vi "Setting.vi"() -> ()   [LabVIEW 2020]
uses:
  Global_Variable/Global.vi
  <userlib>/_MGI/1D Array/MGI Average/MGI Average (DBL[]).vi
  Libraries/S7/S7.lvlib
panel:
  in  "速度":sgl format="%#_3f °/S"
  out "退出":bool=TRUE
  in  "STEP":string
  in  "工位二标定":bool
  in  "停止":bool
  in  "工位一标定":bool
  out "标定曲线":cluster{dbl[], dbl[]}[](graph)
  # "配置标定"
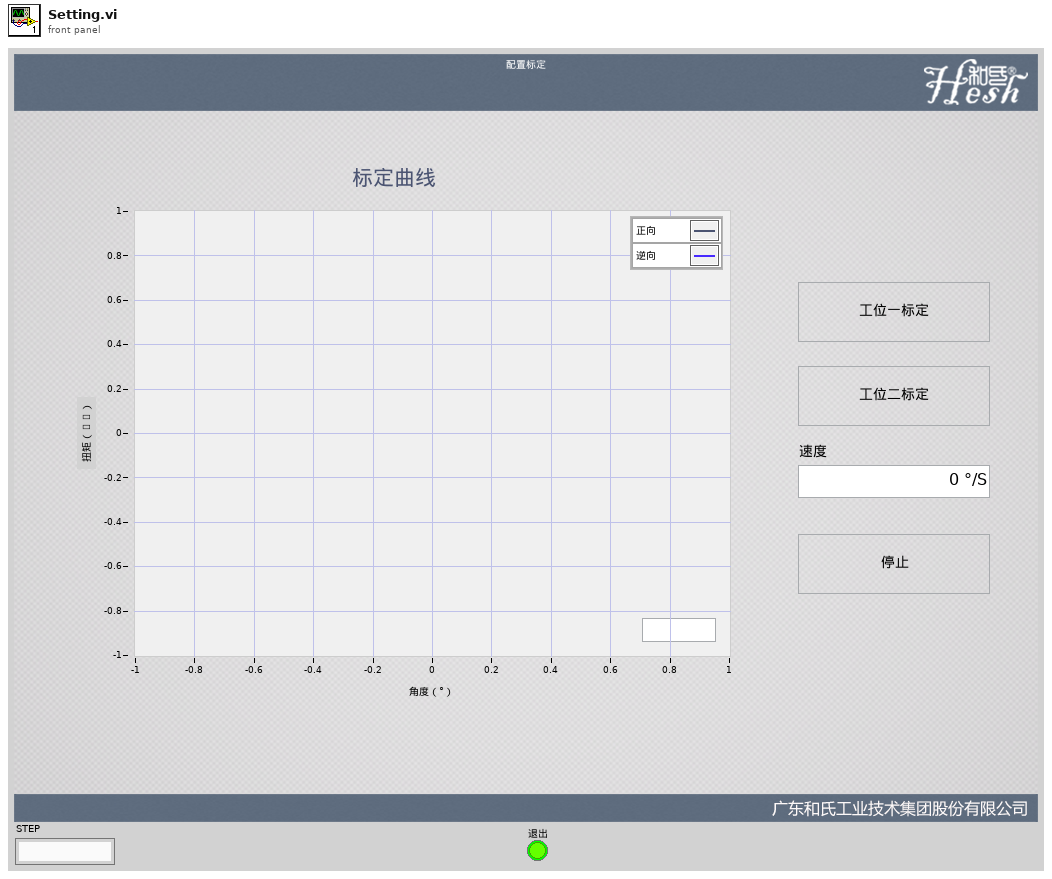
[diagram p1: front panel]
types:
  T1 = cluster{"工位一驱动伺服位移":sgl, "工位二驱动伺服位移":sgl, "工位一移载伺服位移":sgl, "工位二移载伺服位移":sgl, "工位一编码器位移":sgl, "工位二编码器位移":sgl, "工位一扭矩":sgl, "工位二扭矩":sgl}
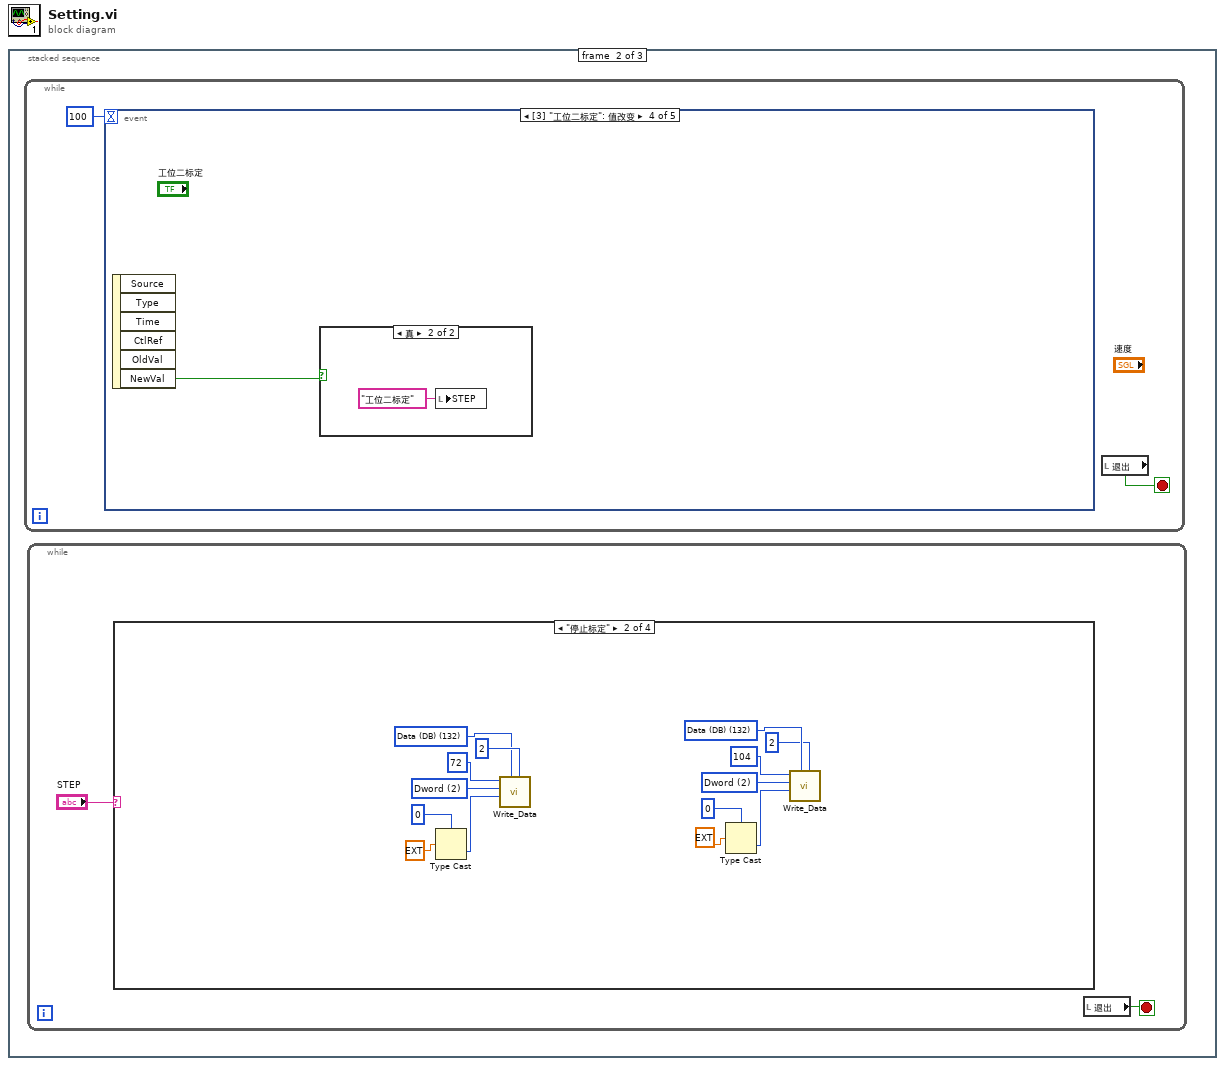
[diagram p0: block diagram]
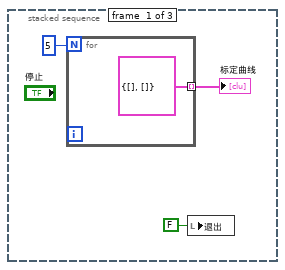
[diagram p2: hidden frame]
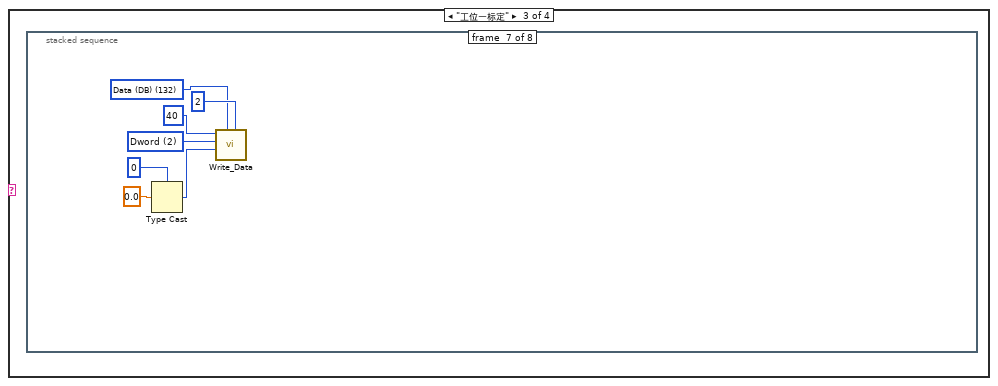
[diagram p4: hidden frame]
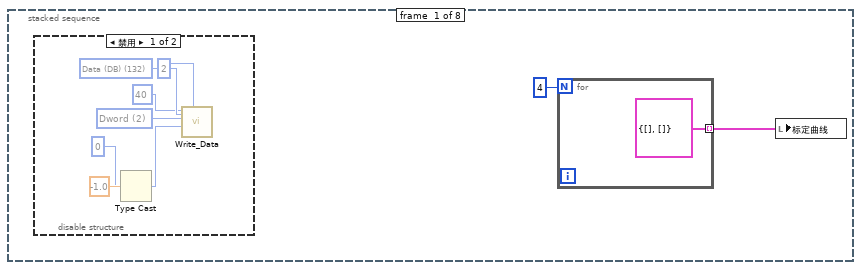
[diagram p5: hidden frame]
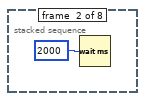
[diagram p7: hidden frame]
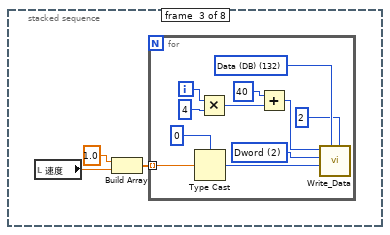
[diagram p8: hidden frame]
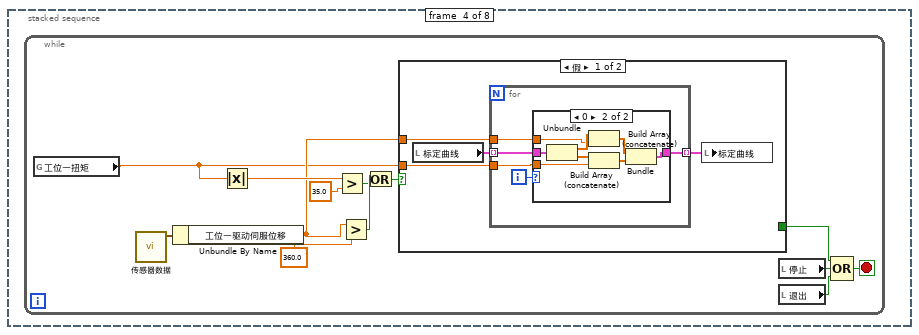
[diagram p9: hidden frame]
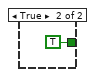
[diagram p11: hidden frame]
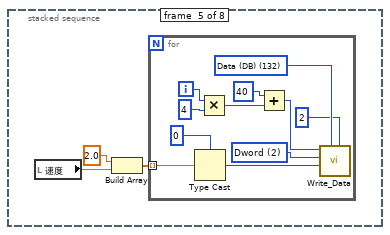
[diagram p12: hidden frame]
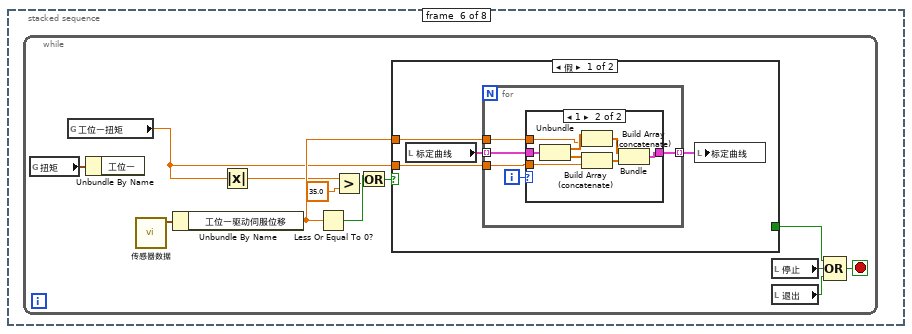
[diagram p13: hidden frame]
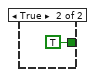
[diagram p15: hidden frame]
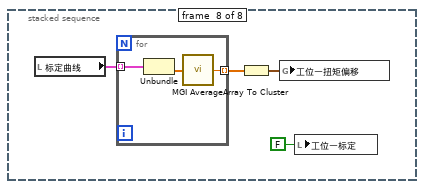
[diagram p16: hidden frame]
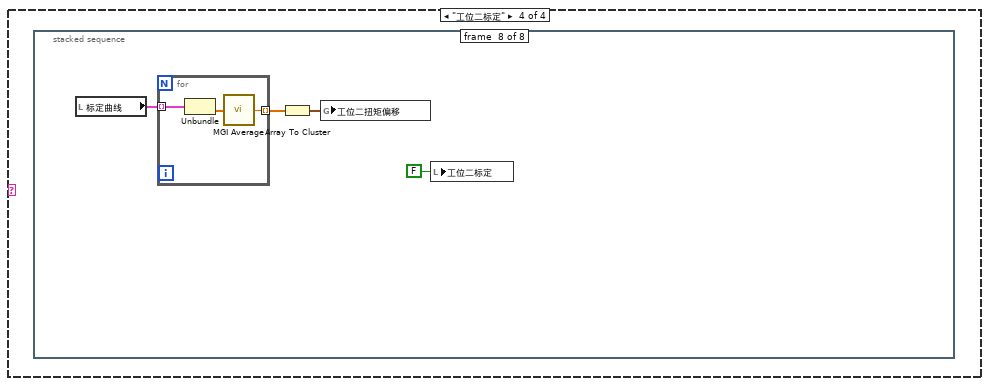
[diagram p17: hidden frame]
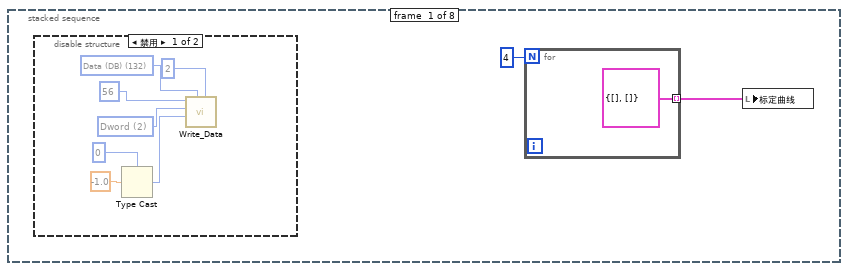
[diagram p18: hidden frame]
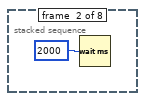
[diagram p20: hidden frame]
diagram:
  n1 = stacked-sequence {
    frame #0 {
      n2 = for {
        N: 5 -> [_]
        tunnel: [cluster{dbl[], dbl[]} {[], []}] -> w2 mode=indexing
      }
      "标定曲线" <- w2
      n3 = local write "退出"(FALSE ("退出")) -> ()
    }
    frame #1 {
      n4 = while {
        stop <- w256 stop-if-true
        n5 = event shown="[3] \"工位二标定\": 值改变" {
          selector: _ -> [_ _ _ _ _]
          dyn-events: _ -> [_ _ _ _ _]
          timeout: 100 -> [_ _ _ _ _]
          event Timeout {
            n6 = event-data() -> ()  [unwired: 1 in, 3 out]
          }
          event "工位一标定": Value Change {
            n7 = event-data() -> ("NewVal"=w258:bool)  [unwired: 1 in, 2 out]
            n8 = case shown="真" w258 {
              frame False {
              }
              frame True {
                n9 = local write "STEP"("工位一标定" ("STEP")) -> ()
              }
            }
          }
          event "停止": Value Change {
            n10 = event-data() -> ()  [unwired: 1 in, 4 out]
            n11 = local write "STEP"("停止标定" ("STEP")) -> ()
          }
          event "工位二标定": Value Change {
            n12 = event-data() -> ("NewVal"=w261:bool)  [unwired: 1 in, 5 out]
            n13 = case shown="真" w261 {
              frame False {
              }
              frame True {
                n14 = local write "STEP"("工位二标定" ("STEP")) -> ()
              }
            }
          }
          event Panel Close {
            n15 = event-data() -> ()  [unwired: 1 in, 4 out]
            n16 = global read "Global.vi" "产品型号"() -> (w264:string)
            n17 = call "标定数据保存.vi"("Section"=w264, "枚举"=enum16{"读取", "保存"}."保存") -> ()  [unwired: 10 in]
            "退出" <- TRUE ("退出")
          }
        }
        n18 = local read "退出"() -> (w256:bool)
      }
      n19 = while {
        stop <- w5 stop-if-true
        n20 = case shown="\"停止标定\"" "STEP" {
          frame "假", Default {
          }
          frame "停止标定" {
            w10 = u16 2 items=["byte", "word", "Dword"] ("数据类型")
            w12 = u8 132 items=["I/O (P)"=128, "Input (I)"=129, "Output (Q)"=130, "Bit Memory (M)"=131, "Data (DB)"=132, "Instance Data (DI)"=133, "Local Data (L)"=134, "Predecessor Local Data (VL)"=135] ("寄存器类型")
            w17 = u16 2 items=["byte", "word", "Dword"] ("数据类型")
            w15 = u8 132 items=["I/O (P)"=128, "Input (I)"=129, "Output (Q)"=130, "Bit Memory (M)"=131, "Data (DB)"=132, "Instance Data (DI)"=133, "Local Data (L)"=134, "Predecessor Local Data (VL)"=135] ("寄存器类型")
            n21 = Type Cast(type=u32 0, x=ext 0.0) -> (*(type *) &x=w19:u32)
            n22 = call "Write_Data.vi"("DB #"=u16 2, "寄存器类型"=w15, "写入数据"=w19, "数据类型"=w17, "写入地址"=u32 72) -> ()  [unwired: 4 in, 3 out]
            n23 = Type Cast(type=u32 0, x=ext 0.0) -> (*(type *) &x=w8:u32)
            n24 = call "Write_Data.vi"("DB #"=u16 2, "寄存器类型"=w12, "写入数据"=w8, "数据类型"=w10, "写入地址"=u32 104) -> ()  [unwired: 4 in, 3 out]
          }
          frame "工位一标定" {
            n25 = stacked-sequence {
              frame #0 {
                n26 = disable-structure shown="禁用" {
                  frame Disabled {
                    w26 = u16 2 items=["byte", "word", "Dword"] ("数据类型")
                    w28 = u8 132 items=["I/O (P)"=128, "Input (I)"=129, "Output (Q)"=130, "Bit Memory (M)"=131, "Data (DB)"=132, "Instance Data (DI)"=133, "Local Data (L)"=134, "Predecessor Local Data (VL)"=135] ("寄存器类型")
                    n27 = Type Cast(type=u32 0, x=sgl -1.0 ("元素")) -> (*(type *) &x=w24:u32)
                    n28 = call "Write_Data.vi"("DB #"=u16 2, "寄存器类型"=w28, "写入数据"=w24, "数据类型"=w26, "写入地址"=u32 40) -> ()  [unwired: 4 in, 3 out]
                  }
                  frame Enabled {
                  }
                }
                n29 = for {
                  N: 4 -> [_]
                  tunnel: [cluster{dbl[], dbl[]} {[], []}] -> w22 mode=indexing
                }
                n30 = local write "标定曲线"(w22) -> ()
              }
              frame #1 {
                n31 = Wait (ms)(milliseconds to wait=u32 2000 ("等待时间（毫秒）")) -> ()  [unwired: 1 out]
              }
              frame #2 {
                n32 = local read "速度"() -> (w32:sgl)
                n33 = Build Array(sgl 1.0 ("元素"), w32) -> (w33:sgl[])
                n34 = for {
                  tunnel: w33 -> [w40] mode=indexing
                  i -> [w37]
                  w42 = u16 2 items=["byte", "word", "Dword"] ("数据类型")
                  w45 = u8 132 items=["I/O (P)"=128, "Input (I)"=129, "Output (Q)"=130, "Bit Memory (M)"=131, "Data (DB)"=132, "Instance Data (DI)"=133, "Local Data (L)"=134, "Predecessor Local Data (VL)"=135] ("寄存器类型")
                  n35 = Type Cast(type=u32 0, x=w40) -> (*(type *) &x=w39:u32)
                  n36 = Multiply(x=w37, y=u32 4) -> (x*y=w36:u32)
                  n37 = Add(x=u32 40 ("写入地址"), y=w36) -> (x+y=w35:u32)
                  n38 = call "Write_Data.vi"("DB #"=u16 2, "寄存器类型"=w45, "写入数据"=w39, "数据类型"=w42, "写入地址"=w35) -> ()  [unwired: 4 in, 3 out]
                }
              }
              frame #3 {
                n39 = while {
                  stop <- w57 stop-if-true
                  n40 = global read "Global.vi" "工位一扭矩"() -> (w46:dbl)
                  n41 = call "传感器数据.vi"() -> ("传感器读数"=w58:T1)  [unwired: 11 in]
                  n42 = Unbundle By Name(w58) -> ("工位一驱动伺服位移"=w48:sgl)
                  n43 = Absolute Value(x=w46) -> (abs(x)=w54:dbl)
                  n44 = Greater?(x=w54, y=35.0) -> (0:w51:bool)
                  n45 = Greater?(x=w48, y=sgl 360.0) -> (0:w52:bool)
                  n46 = Or(x=w52, y=w51) -> (x .or. y?=w50:bool)
                  n47 = case shown="假" w50 {
                    tunnel: [_ TRUE] -> w56
                    tunnel: w48 -> [w61 _]
                    tunnel: w46 -> [w60 _]
                    frame False {
                      n48 = local read "标定曲线"() -> (w62:cluster{dbl[], dbl[]}[])
                      n49 = for {
                        tunnel: w62 -> [w67] mode=indexing
                        tunnel: w61 -> [w66]
                        tunnel: w60 -> [w65]
                        tunnel: [w63] -> w59 mode=indexing
                        i -> [w64]
                        n50 = case shown="0" w64 {
                          tunnel: w67 -> [w68 w76]
                          tunnel: w66 -> [_ w73]
                          tunnel: w65 -> [_ w72]
                          tunnel: [w68 w69] -> w63
                          frame Default {
                          }
                          frame 0 {
                            n51 = Unbundle(w76) -> (w74:dbl[], w75:dbl[])
                            n52 = Build Array (concatenate)(w74, w73) -> (w71:dbl[])
                            n53 = Build Array (concatenate)(w75, w72) -> (w70:dbl[])
                            n54 = Bundle(w71, w70) -> (w69:cluster{dbl[], dbl[]})  [unwired: 1 in]
                          }
                        }
                      }
                      n55 = local write "标定曲线"(w59) -> ()
                    }
                    frame True {
                    }
                  }
                  n56 = local read "停止"() -> (w55:bool)
                  n57 = local read "退出"() -> (w49:bool)
                  n58 = Compound Arithmetic op=OR ("复合运算")(w56, w55, w49) -> (w57:bool)
                }
              }
              frame #4 {
                n59 = local read "速度"() -> (w78:sgl)
                n60 = Build Array(sgl 2.0 ("元素"), w78) -> (w79:sgl[])
                n61 = for {
                  tunnel: w79 -> [w86] mode=indexing
                  i -> [w83]
                  w88 = u16 2 items=["byte", "word", "Dword"] ("数据类型")
                  w91 = u8 132 items=["I/O (P)"=128, "Input (I)"=129, "Output (Q)"=130, "Bit Memory (M)"=131, "Data (DB)"=132, "Instance Data (DI)"=133, "Local Data (L)"=134, "Predecessor Local Data (VL)"=135] ("寄存器类型")
                  n62 = Type Cast(type=u32 0, x=w86) -> (*(type *) &x=w85:u32)
                  n63 = Multiply(x=w83, y=u32 4) -> (x*y=w82:u32)
                  n64 = Add(x=u32 40 ("写入地址"), y=w82) -> (x+y=w81:u32)
                  n65 = call "Write_Data.vi"("DB #"=u16 2, "寄存器类型"=w91, "写入数据"=w85, "数据类型"=w88, "写入地址"=w81) -> ()  [unwired: 4 in, 3 out]
                }
              }
              frame #5 {
                n66 = while {
                  stop <- w103 stop-if-true
                  n67 = global read "Global.vi" "扭矩"() -> (w99:cluster{"工位一":dbl, "工位二":dbl})
                  n68 = global read "Global.vi" "工位一扭矩"() -> (w92:dbl)
                  n69 = Unbundle By Name(w99) -> ()  [unwired: 1 out]
                  n70 = call "传感器数据.vi"() -> ("传感器读数"=w104:T1)  [unwired: 11 in]
                  n71 = Unbundle By Name(w104) -> ("工位一驱动伺服位移"=w100:sgl)
                  n72 = Absolute Value(x=w92) -> (abs(x)=w98:dbl)
                  n73 = Less Or Equal To 0?(x=w100) -> (x <= 0?=w96:bool)
                  n74 = Greater?(x=w98, y=35.0) -> (0:w95:bool)
                  n75 = Or(x=w96, y=w95) -> (x .or. y?=w94:bool)
                  n76 = case shown="假" w94 {
                    tunnel: [_ TRUE] -> w102
                    tunnel: w100 -> [w107 _]
                    tunnel: w92 -> [w106 _]
                    frame False {
                      n77 = local read "标定曲线"() -> (w108:cluster{dbl[], dbl[]}[])
                      n78 = for {
                        tunnel: w108 -> [w113] mode=indexing
                        tunnel: w107 -> [w112]
                        tunnel: w106 -> [w111]
                        tunnel: [w109] -> w105 mode=indexing
                        i -> [w110]
                        n79 = case shown="1" w110 {
                          tunnel: w113 -> [w114 w122]
                          tunnel: w112 -> [_ w119]
                          tunnel: w111 -> [_ w118]
                          tunnel: [w114 w115] -> w109
                          frame Default {
                          }
                          frame 1 {
                            n80 = Unbundle(w122) -> (w120:dbl[], w121:dbl[])
                            n81 = Build Array (concatenate)(w120, w119) -> (w117:dbl[])
                            n82 = Build Array (concatenate)(w121, w118) -> (w116:dbl[])
                            n83 = Bundle(w117, w116) -> (w115:cluster{dbl[], dbl[]})  [unwired: 1 in]
                          }
                        }
                      }
                      n84 = local write "标定曲线"(w105) -> ()
                    }
                    frame True {
                    }
                  }
                  n85 = local read "停止"() -> (w101:bool)
                  n86 = local read "退出"() -> (w93:bool)
                  n87 = Compound Arithmetic op=OR ("复合运算")(w102, w101, w93) -> (w103:bool)
                }
              }
              frame #6 {
                w127 = u16 2 items=["byte", "word", "Dword"] ("数据类型")
                w125 = u8 132 items=["I/O (P)"=128, "Input (I)"=129, "Output (Q)"=130, "Bit Memory (M)"=131, "Data (DB)"=132, "Instance Data (DI)"=133, "Local Data (L)"=134, "Predecessor Local Data (VL)"=135] ("寄存器类型")
                n88 = Type Cast(type=u32 0, x=sgl 0.0) -> (*(type *) &x=w129:u32)
                n89 = call "Write_Data.vi"("DB #"=u16 2, "寄存器类型"=w125, "写入数据"=w129, "数据类型"=w127, "写入地址"=u32 40) -> ()  [unwired: 4 in, 3 out]
              }
              frame #7 {
                n90 = local read "标定曲线"() -> (w134:cluster{dbl[], dbl[]}[])
                n91 = for {
                  tunnel: w134 -> [w137] mode=indexing
                  tunnel: [w135] -> w133 mode=indexing
                  n92 = Unbundle(w137) -> (w136:dbl[])  [unwired: 1 out]
                  n93 = call-poly <userlib>:"MGI Average.vi"("Double[]"=w136) -> ("Average"=w135:dbl)  [unwired: 1 in]
                }
                n94 = Array To Cluster(array=w133) -> (cluster=w132:cluster{"[0]":dbl, "[1]":dbl})
                n95 = global write "Global.vi" "工位一扭矩偏移"(w132) -> ()
                n96 = local write "工位一标定"(FALSE ("工位一标定")) -> ()
              }
            }
          }
          frame "工位二标定" {
            n97 = stacked-sequence {
              frame #0 {
                n98 = disable-structure shown="禁用" {
                  frame Disabled {
                    w143 = u16 2 items=["byte", "word", "Dword"] ("数据类型")
                    w145 = u8 132 items=["I/O (P)"=128, "Input (I)"=129, "Output (Q)"=130, "Bit Memory (M)"=131, "Data (DB)"=132, "Instance Data (DI)"=133, "Local Data (L)"=134, "Predecessor Local Data (VL)"=135] ("寄存器类型")
                    n99 = Type Cast(type=u32 0, x=sgl -1.0 ("元素")) -> (*(type *) &x=w141:u32)
                    n100 = call "Write_Data.vi"("DB #"=u16 2, "寄存器类型"=w145, "写入数据"=w141, "数据类型"=w143, "写入地址"=u32 56) -> ()  [unwired: 4 in, 3 out]
                  }
                  frame Enabled {
                  }
                }
                n101 = for {
                  N: 4 -> [_]
                  tunnel: [cluster{dbl[], dbl[]} {[], []}] -> w139 mode=indexing
                }
                n102 = local write "标定曲线"(w139) -> ()
              }
              frame #1 {
                n103 = Wait (ms)(milliseconds to wait=u32 2000 ("等待时间（毫秒）")) -> ()  [unwired: 1 out]
              }
              frame #2 {
                n104 = local read "速度"() -> (w149:sgl)
                n105 = Build Array(sgl 1.0 ("元素"), w149) -> (w150:sgl[])
                n106 = for {
                  tunnel: w150 -> [w157] mode=indexing
                  i -> [w154]
                  w159 = u16 2 items=["byte", "word", "Dword"] ("数据类型")
                  w162 = u8 132 items=["I/O (P)"=128, "Input (I)"=129, "Output (Q)"=130, "Bit Memory (M)"=131, "Data (DB)"=132, "Instance Data (DI)"=133, "Local Data (L)"=134, "Predecessor Local Data (VL)"=135] ("寄存器类型")
                  n107 = Type Cast(type=u32 0, x=w157) -> (*(type *) &x=w156:u32)
                  n108 = Multiply(x=w154, y=u32 4) -> (x*y=w153:u32)
                  n109 = Add(x=u32 56 ("写入地址"), y=w153) -> (x+y=w152:u32)
                  n110 = call "Write_Data.vi"("DB #"=u16 2, "寄存器类型"=w162, "写入数据"=w156, "数据类型"=w159, "写入地址"=w152) -> ()  [unwired: 4 in, 3 out]
                }
              }
              frame #3 {
                n111 = while {
                  stop <- w175 stop-if-true
                  n112 = global read "Global.vi" "扭矩"() -> (w172:cluster{"工位一":dbl, "工位二":dbl})
                  n113 = Unbundle By Name(w172) -> ()  [unwired: 1 out]
                  n114 = global read "Global.vi" "工位二扭矩"() -> (w163:dbl)
                  n115 = call "传感器数据.vi"() -> ("传感器读数"=w176:T1)  [unwired: 11 in]
                  n116 = Unbundle By Name(w176) -> ("工位二驱动伺服位移"=w165:sgl)
                  n117 = Absolute Value(x=w163) -> (abs(x)=w171:dbl)
                  n118 = Greater?(x=w171, y=35.0) -> (0:w168:bool)
                  n119 = Greater?(x=w165, y=sgl 360.0) -> (0:w169:bool)
                  n120 = Or(x=w169, y=w168) -> (x .or. y?=w167:bool)
                  n121 = case shown="假" w167 {
                    tunnel: [_ TRUE] -> w174
                    tunnel: w165 -> [w179 _]
                    tunnel: w163 -> [w178 _]
                    frame False {
                      n122 = local read "标定曲线"() -> (w180:cluster{dbl[], dbl[]}[])
                      n123 = for {
                        tunnel: w180 -> [w185] mode=indexing
                        tunnel: w179 -> [w184]
                        tunnel: w178 -> [w183]
                        tunnel: [w181] -> w177 mode=indexing
                        i -> [w182]
                        n124 = case shown="默认" w182 {
                          tunnel: w185 -> [w186 w194]
                          tunnel: w184 -> [_ w191]
                          tunnel: w183 -> [_ w190]
                          tunnel: [w186 w187] -> w181
                          frame Default {
                          }
                          frame 0 {
                            n125 = Unbundle(w194) -> (w192:dbl[], w193:dbl[])
                            n126 = Build Array (concatenate)(w192, w191) -> (w189:dbl[])
                            n127 = Build Array (concatenate)(w193, w190) -> (w188:dbl[])
                            n128 = Bundle(w189, w188) -> (w187:cluster{dbl[], dbl[]})  [unwired: 1 in]
                          }
                        }
                      }
                      n129 = local write "标定曲线"(w177) -> ()
                    }
                    frame True {
                    }
                  }
                  n130 = local read "停止"() -> (w173:bool)
                  n131 = local read "退出"() -> (w166:bool)
                  n132 = Compound Arithmetic op=OR ("复合运算")(w174, w173, w166) -> (w175:bool)
                }
              }
              frame #4 {
                n133 = local read "速度"() -> (w196:sgl)
                n134 = Build Array(sgl 2.0 ("元素"), w196) -> (w197:sgl[])
                n135 = for {
                  tunnel: w197 -> [w204] mode=indexing
                  i -> [w201]
                  w206 = u16 2 items=["byte", "word", "Dword"] ("数据类型")
                  w209 = u8 132 items=["I/O (P)"=128, "Input (I)"=129, "Output (Q)"=130, "Bit Memory (M)"=131, "Data (DB)"=132, "Instance Data (DI)"=133, "Local Data (L)"=134, "Predecessor Local Data (VL)"=135] ("寄存器类型")
                  n136 = Type Cast(type=u32 0, x=w204) -> (*(type *) &x=w203:u32)
                  n137 = Multiply(x=w201, y=u32 4) -> (x*y=w200:u32)
                  n138 = Add(x=u32 56 ("写入地址"), y=w200) -> (x+y=w199:u32)
                  n139 = call "Write_Data.vi"("DB #"=u16 2, "寄存器类型"=w209, "写入数据"=w203, "数据类型"=w206, "写入地址"=w199) -> ()  [unwired: 4 in, 3 out]
                }
              }
              frame #5 {
                n140 = while {
                  stop <- w221 stop-if-true
                  n141 = global read "Global.vi" "扭矩"() -> (w217:cluster{"工位一":dbl, "工位二":dbl})
                  n142 = global read "Global.vi" "工位二扭矩"() -> (w210:dbl)
                  n143 = Unbundle By Name(w217) -> ()  [unwired: 1 out]
                  n144 = call "传感器数据.vi"() -> ("传感器读数"=w222:T1)  [unwired: 11 in]
                  n145 = Unbundle By Name(w222) -> ("工位二驱动伺服位移"=w218:sgl)
                  n146 = Absolute Value(x=w210) -> (abs(x)=w216:dbl)
                  n147 = Less Or Equal To 0?(x=w218) -> (x <= 0?=w214:bool)
                  n148 = Greater?(x=w216, y=35.0) -> (0:w213:bool)
                  n149 = Or(x=w214, y=w213) -> (x .or. y?=w212:bool)
                  n150 = case shown="假" w212 {
                    tunnel: [_ TRUE] -> w220
                    tunnel: w218 -> [w225 _]
                    tunnel: w210 -> [w224 _]
                    frame False {
                      n151 = local read "标定曲线"() -> (w226:cluster{dbl[], dbl[]}[])
                      n152 = for {
                        tunnel: w226 -> [w231] mode=indexing
                        tunnel: w225 -> [w230]
                        tunnel: w224 -> [w229]
                        tunnel: [w227] -> w223 mode=indexing
                        i -> [w228]
                        n153 = case shown="1" w228 {
                          tunnel: w231 -> [w232 w240]
                          tunnel: w230 -> [_ w237]
                          tunnel: w229 -> [_ w236]
                          tunnel: [w232 w233] -> w227
                          frame Default {
                          }
                          frame 1 {
                            n154 = Unbundle(w240) -> (w238:dbl[], w239:dbl[])
                            n155 = Build Array (concatenate)(w238, w237) -> (w235:dbl[])
                            n156 = Build Array (concatenate)(w239, w236) -> (w234:dbl[])
                            n157 = Bundle(w235, w234) -> (w233:cluster{dbl[], dbl[]})  [unwired: 1 in]
                          }
                        }
                      }
                      n158 = local write "标定曲线"(w223) -> ()
                    }
                    frame True {
                    }
                  }
                  n159 = local read "停止"() -> (w219:bool)
                  n160 = local read "退出"() -> (w211:bool)
                  n161 = Compound Arithmetic op=OR ("复合运算")(w220, w219, w211) -> (w221:bool)
                }
              }
              frame #6 {
                w245 = u16 2 items=["byte", "word", "Dword"] ("数据类型")
                w246 = u8 132 items=["I/O (P)"=128, "Input (I)"=129, "Output (Q)"=130, "Bit Memory (M)"=131, "Data (DB)"=132, "Instance Data (DI)"=133, "Local Data (L)"=134, "Predecessor Local Data (VL)"=135] ("寄存器类型")
                n162 = Type Cast(type=u32 0, x=sgl 0.0) -> (*(type *) &x=w248:u32)
                n163 = call "Write_Data.vi"("DB #"=u16 2, "寄存器类型"=w246, "写入数据"=w248, "数据类型"=w245, "写入地址"=u32 56) -> ()  [unwired: 4 in, 3 out]
              }
              frame #7 {
                n164 = local read "标定曲线"() -> (w252:cluster{dbl[], dbl[]}[])
                n165 = for {
                  tunnel: w252 -> [w255] mode=indexing
                  tunnel: [w253] -> w251 mode=indexing
                  n166 = Unbundle(w255) -> (w254:dbl[])  [unwired: 1 out]
                  n167 = call-poly <userlib>:"MGI Average.vi"("Double[]"=w254) -> ("Average"=w253:dbl)  [unwired: 1 in]
                }
                n168 = Array To Cluster(array=w251) -> (cluster=w250:cluster{"[0]":dbl, "[1]":dbl})
                n169 = global write "Global.vi" "工位二扭矩偏移"(w250) -> ()
                n170 = local write "工位二标定"(FALSE ("工位一标定")) -> ()
              }
            }
          }
        }
        n171 = local read "退出"() -> (w5:bool)
      }
    }
    frame #2 {
      w269 = u16 2 items=["byte", "word", "Dword"] ("数据类型")
      w271 = u8 132 items=["I/O (P)"=128, "Input (I)"=129, "Output (Q)"=130, "Bit Memory (M)"=131, "Data (DB)"=132, "Instance Data (DI)"=133, "Local Data (L)"=134, "Predecessor Local Data (VL)"=135] ("寄存器类型")
      w276 = u16 2 items=["byte", "word", "Dword"] ("数据类型")
      w274 = u8 132 items=["I/O (P)"=128, "Input (I)"=129, "Output (Q)"=130, "Bit Memory (M)"=131, "Data (DB)"=132, "Instance Data (DI)"=133, "Local Data (L)"=134, "Predecessor Local Data (VL)"=135] ("寄存器类型")
      n172 = Type Cast(type=u32 0, x=sgl 0.0) -> (*(type *) &x=w278:u32)
      n173 = call "Write_Data.vi"("DB #"=u16 2, "寄存器类型"=w274, "写入数据"=w278, "数据类型"=w276, "写入地址"=u32 72) -> ()  [unwired: 4 in, 3 out]
      n174 = Type Cast(type=u32 0, x=sgl 0.0) -> (*(type *) &x=w267:u32)
      n175 = call "Write_Data.vi"("DB #"=u16 2, "寄存器类型"=w271, "写入数据"=w267, "数据类型"=w269, "写入地址"=u32 104) -> ()  [unwired: 4 in, 3 out]
    }
  }
